vi "FPGA_GetRef.vi"(2 "error in (no error)":errorcluster) -> (0 "error out":errorcluster, 1 "FPGA_Ref":refnum<k20>)   [LabVIEW 2009, in "FPGA.lvlib"]
doc: "Returns the reference to an open FPGA. Need to be called in between FPGA_Open and FPGA_Close."
uses:
  FPGA.lvlib
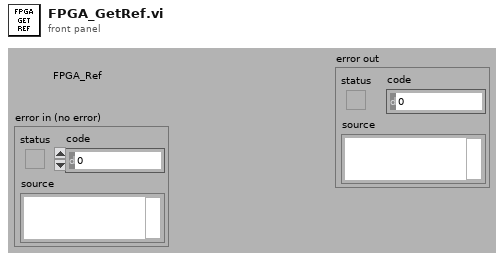
[diagram p1: front panel]
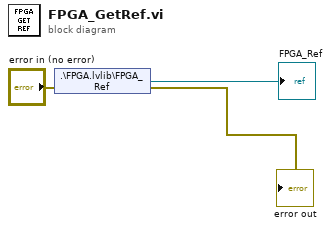
[diagram p0: block diagram]
diagram:
  n1 = shared-variable ".\\FPGA.lvlib\\FPGA_Ref"(error in="error in (no error)") -> (→"FPGA_Ref":refnum<k20>, error out=→"error out":errorcluster)
